vi "Restore Offset to Tilted Logistic Square Pulse Parameters.vi"(8 "Error In":errorcluster, 9 "Offset":dbl, 11 "Best Fit Parameters":dbl[](array[numeric])) -> (0 "Error Out":errorcluster, 3 "Offset Best Fit Parameters":dbl[](array[numeric]))   [LabVIEW 2021, in "Fits.lvlib"]
uses:
  Fits.lvlib
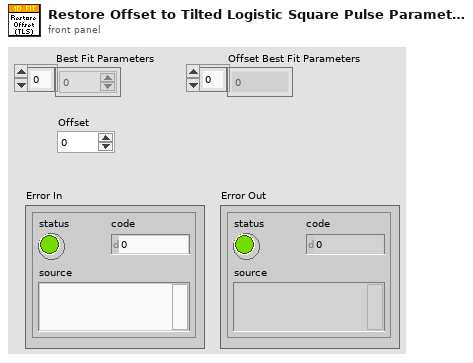
[diagram p1: front panel]
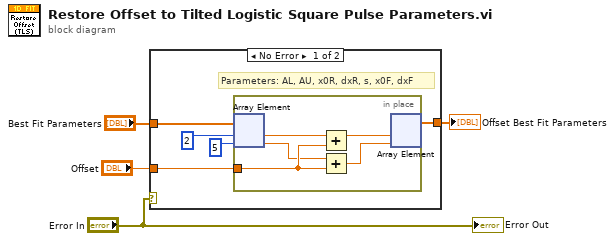
[diagram p0: block diagram]
diagram:
  n1 = case shown="No Error" "Error In" {
    tunnel: "Offset" -> [w9 _]
    tunnel: "Best Fit Parameters" -> [w8 w15]
    tunnel: [w7 w15] -> w2
    frame No Error {
      # "Parameters: AL, AU, x0R, dxR, s, x0F, dxF"
      n2 = in-place {
        in-place-border: w9 -> [w14]
        n3 = in-place-array #1(w8, 2, 5) -> (w13:dbl, w11:dbl)
        n4 = Add(x=w13, y=w14) -> (x+y=w12:dbl)
        n5 = Add(x=w11, y=w14) -> (x+y=w10:dbl)
        n6 = in-place-array #1(w12, w10) -> (w7:dbl[])  [unwired: 2 out]
      }
    }
    frame Error {
    }
  }
  "Offset Best Fit Parameters" <- w2
  "Error Out" <- "Error In"
